vi "Listen to RPi.vi"(8 "error in (no error)":errorcluster, 11 "port":u16) -> (0 "error out":errorcluster, 3 "data out":string)   [LabVIEW 2016, in "Huskie Swerve.lvlib"]
uses:
  Huskie Swerve.lvlib
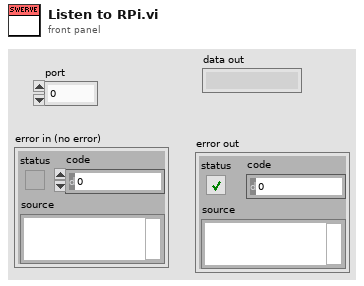
[diagram p1: front panel]
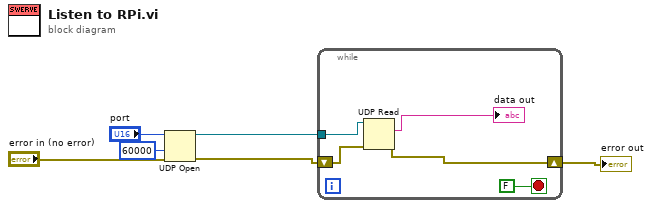
[diagram p0: block diagram]
diagram:
  n1 = UDP Open(8:"error in (no error)", 9:60000 ("timeout ms (25000)"), 11:"port") -> (port=w2:refnum<k16>, 0:w4:errorcluster)  [unwired: 2 in, 1 out]
  n2 = while {
    shift-right: [w7] -> w1
    shift-left: w4 -> [w8]
    tunnel: w2 -> [w10]
    stop <- FALSE stop-if-true
    n3 = UDP Read(connection ID=w10, 8:w8) -> (data out=→"data out":string, error out=w7:errorcluster)  [unwired: 2 in, 3 out]
  }
  "error out" <- w1
